vi "GetSwerveEncoders.vi"() -> (20 "Swerve 0 Azimuth Position (deg)":dbl, 21 "Swerve 0 Distance (in)":dbl, 22 "Swerve 1 Azimuth Position (deg)":dbl, 23 "Swerve 1 Distance (in)":dbl, 24 "Swerve 2 Azimuth Position (deg)":dbl, 25 "Swerve 2 Distance (in)":dbl, 26 "Swerve 3 Azimuth Position (deg)":dbl, 27 "Swerve 3 Distance (in)":dbl)   [LabVIEW 2019]
doc: "Gets the drive distance, azimuth position, and velocity encoder readings from the swerve."
uses:
  refnums.vi
  GRNF_POT.vi
  dsdata.vi
  <vilib>/Utility/xml.llb/Write to XML File(string).vi
  outputs.vi
  sensors.vi
  GRNF_CTREMotor.vi
  <vilib>/Rock Robotics/WPI/ThirdParty/Phoenix-LabVIEW/Motor Controller/Get/CTRE_Phoenix_MotorController_GetSelectedSensorData.vi
panel:
  in  "Plot":bool
  out "Drive Encoder Velocities":cluster{dbl, dbl, dbl, dbl}(graph)
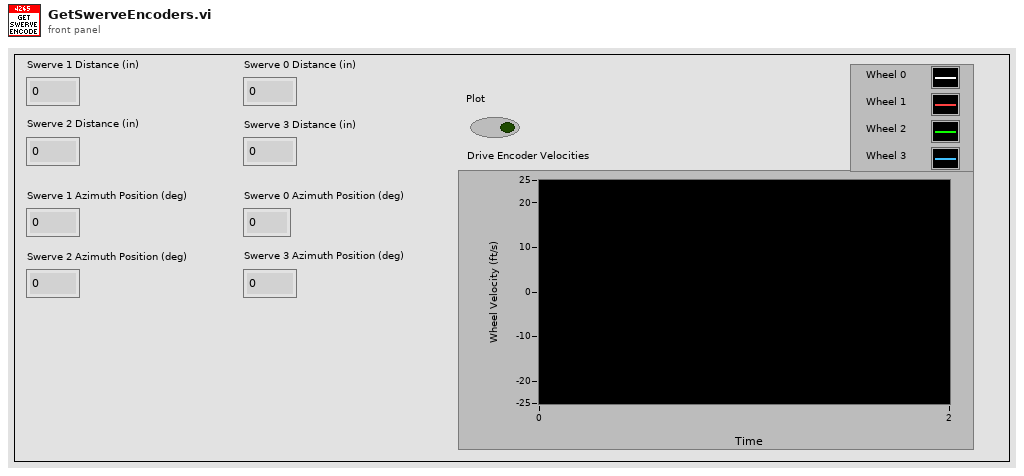
[diagram p1: front panel]
types:
  T1 = typedef "WPI_MotorControlDeviceRef.ctl" = cluster{"DeviceStatus":errorcluster, "Type":T2, "PWM":cluster{"PWM Channel":T3, "DeadBand":T4}, "CAN":cluster{"Device Number":u8, "SetOutput VI Ref":variant, "GetOutput VI Ref":variant, "Enable VI Ref":variant, "Disable VI Ref":variant, "Data":variant}, "Invert":bool, "DIO PWM":cluster{"PWM \"Enable\" Channel":T3, "DIOChannel":T5, "PWM Rate":dbl}}
  T2 = typedef "WPI_MotorControlType.ctl" = enum16{"PWM", "CAN", "DIO PWM"}
  T3 = typedef "FPGA_DIOPWMChannel.ctl" = enum8{"PWM 0", "PWM 1", "PWM 2", "PWM 3", "PWM 4", "PWM 5", "PWM 6", "PWM 7", "PWM 8", "PWM 9", "PWM MXP 0", "PWM MXP 1", "PWM MXP 2", "PWM MXP 3", "PWM MXP 4", "PWM MXP 5", "PWM MXP 6", "PWM MXP 7", "PWM MXP 8", "PWM MXP 9", "Invalid"}
  T4 = typedef "WPI_PWMDeadband.ctl" = cluster{"Name":string, "maxPositivePwm":i32, "minPositivePwm":i32, "centerPwm":i32, "maxNegativePwm":i32, "minNegativePwm":i32, "angularRange":u16}
  T5 = typedef "FPGA_DIOChannel.ctl" = enum8{"DIO 0", "DIO 1", "DIO 2", "DIO 3", "DIO 4", "DIO 5", "DIO 6", "DIO 7", "DIO 8", "DIO 9", "DIO MXP 0", "DIO MXP 1", "DIO MXP 2", "DIO MXP 3", "DIO MXP 4", "DIO MXP 5", "DIO MXP 6", "DIO MXP 7", "DIO MXP 8", "DIO MXP 9", "DIO MXP 10", "DIO MXP 11", "DIO MXP 12", "DIO MXP 13", "DIO MXP 14", "DIO MXP 15", "SPI Port CS1", "SPI Port CS2", "SPI Port CS3", "SPI Port MISO", "SPI Port MOSI", "Invalid"}
  T6 = typedef "WPI_PotentiometerDevRef.ctl" = cluster{"DevStatus":errorcluster, "Analog Channel":T7, "Invert Output":bool}
  T7 = typedef "FPGA_AIChannel.ctl" = enum8{"AI 0", "AI 1", "AI 2", "AI 3", "AI MXP 0", "AI MXP 1", "AI MXP 2", "AI MXP 3", "Invalid"}
  T8 = cluster{"Command Output":bool, "Time Output (ms)":u32}
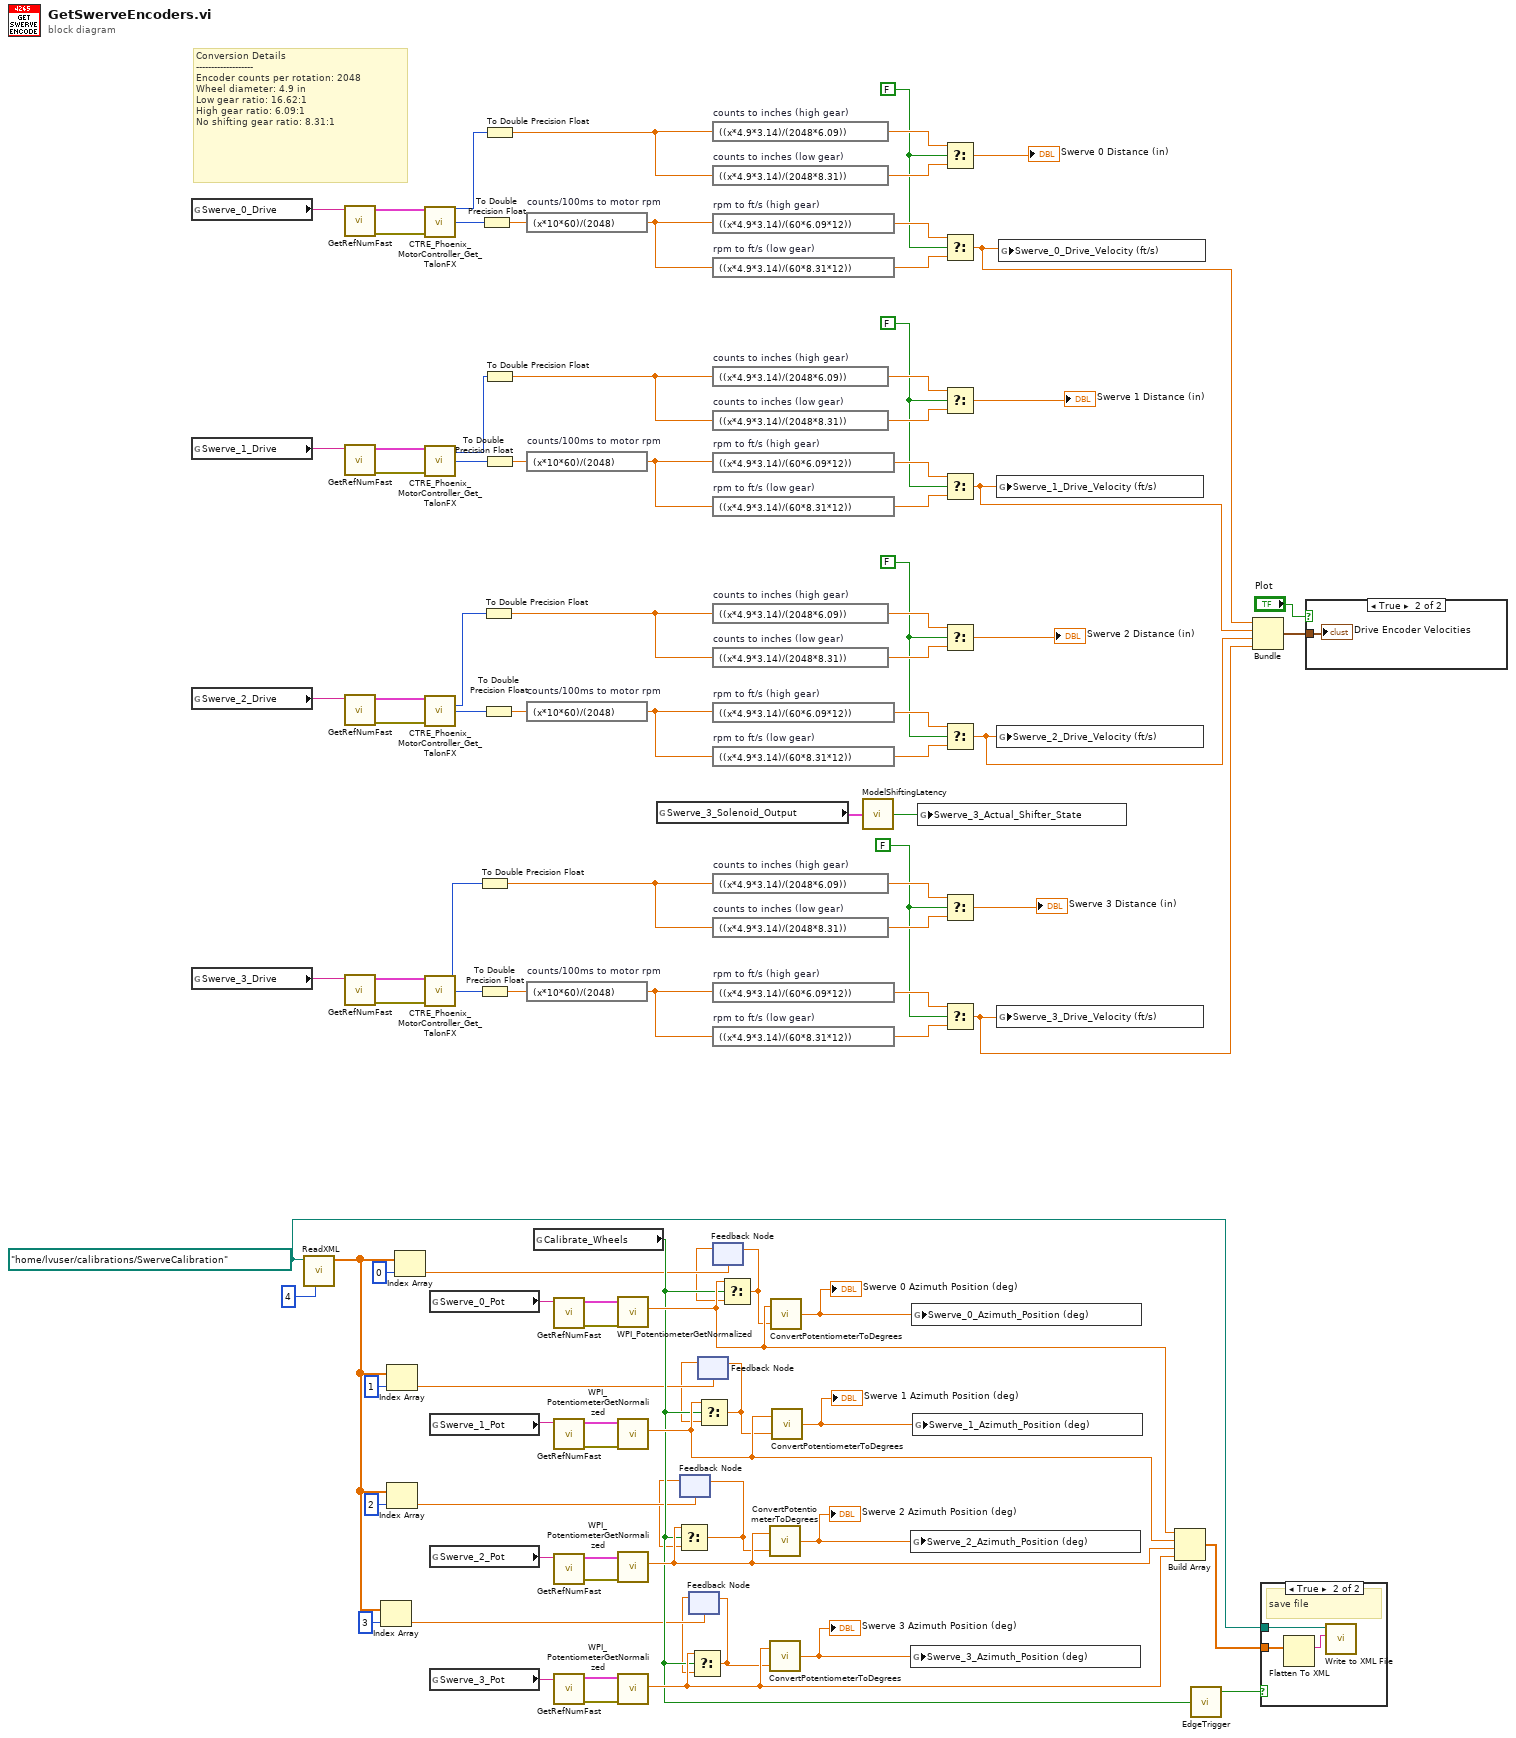
[diagram p0: block diagram]
diagram:
  w13 = FALSE
  w15 = FALSE
  w16 = FALSE
  w17 = FALSE
  w101 = path "/home/lvuser/calibrations/SwerveCalibration" ("path")
  # "Conversion Details\n-------------------\nEncoder counts per rotation: 2048\nWheel diameter: 4.9 in\nLow gear ratio: 16.62:1\nHigh gear ratio: 6.09:1\nNo shifting gear ratio: 8.31:1"
  n1 = global read "refnums.vi" "Swerve_0_Drive"() -> (w25:string)
  n2 = global read "refnums.vi" "Swerve_1_Drive"() -> (w36:string)
  n3 = global read "refnums.vi" "Swerve_2_Drive"() -> (w48:string)
  n4 = global read "refnums.vi" "Swerve_3_Drive"() -> (w58:string)
  n5 = call "ReadXML.vi"("Default Number of Elements"=4 ("Number of Elements"), "File Path (.xml)"=w101) -> ("Data"=w66:dbl[])  [unwired: 8 in, 1 out]
  n6 = call-poly "GetRefNumFast.vi"("RefNum Name"=w25) -> ("Error"=w27:errorcluster, "Device Reference"=w26:T1)  [unwired: 5 in]
  n7 = call-poly "GetRefNumFast.vi"("RefNum Name"=w36) -> ("Error"=w38:errorcluster, "Device Reference"=w37:T1)  [unwired: 5 in]
  n8 = call-poly "GetRefNumFast.vi"("RefNum Name"=w48) -> ("Error"=w50:errorcluster, "Device Reference"=w49:T1)  [unwired: 5 in]
  n9 = call-poly "GetRefNumFast.vi"("RefNum Name"=w58) -> ("Error"=w60:errorcluster, "Device Reference"=w59:T1)  [unwired: 5 in]
  n10 = Index Array(array=w66, index=3) -> (element=w85:dbl)
  n11 = Index Array(array=w66, index=1) -> (element=w90:dbl)
  n12 = Index Array(array=w66, index=2) -> (element=w87:dbl)
  n13 = Index Array(array=w66, index=0) -> (element=w93:dbl)
  n14 = call-poly <vilib>:"CTRE_Phoenix_MotorController_Get_TalonFX.vi"("PhoenixMotorControlDevRef"=w26, "error in"=w27) -> ("Position (Raw Sensor Units)"=w19:i32, "Velocity (Raw Sensor Units per 100 ms)"=w21:i32)  [unwired: 10 in, 2 out]
  n15 = call-poly <vilib>:"CTRE_Phoenix_MotorController_Get_TalonFX.vi"("PhoenixMotorControlDevRef"=w37, "error in"=w38) -> ("Position (Raw Sensor Units)"=w30:i32, "Velocity (Raw Sensor Units per 100 ms)"=w32:i32)  [unwired: 10 in, 2 out]
  n16 = call-poly <vilib>:"CTRE_Phoenix_MotorController_Get_TalonFX.vi"("PhoenixMotorControlDevRef"=w49, "error in"=w50) -> ("Position (Raw Sensor Units)"=w42:i32, "Velocity (Raw Sensor Units per 100 ms)"=w44:i32)  [unwired: 10 in, 2 out]
  n17 = call-poly <vilib>:"CTRE_Phoenix_MotorController_Get_TalonFX.vi"("PhoenixMotorControlDevRef"=w59, "error in"=w60) -> ("Position (Raw Sensor Units)"=w52:i32, "Velocity (Raw Sensor Units per 100 ms)"=w54:i32)  [unwired: 10 in, 2 out]
  n18 = global read "refnums.vi" "Swerve_0_Pot"() -> (w78:string)
  n19 = global read "refnums.vi" "Swerve_1_Pot"() -> (w73:string)
  n20 = global read "refnums.vi" "Swerve_2_Pot"() -> (w70:string)
  n21 = global read "refnums.vi" "Swerve_3_Pot"() -> (w69:string)
  n22 = To Double Precision Float(number=w52) -> (double precision float=w12:dbl)
  n23 = To Double Precision Float(number=w54) -> (double precision float=w11:dbl)
  n24 = To Double Precision Float(number=w21) -> (double precision float=w5:dbl)
  n25 = To Double Precision Float(number=w42) -> (double precision float=w10:dbl)
  n26 = To Double Precision Float(number=w44) -> (double precision float=w9:dbl)
  n27 = To Double Precision Float(number=w19) -> (double precision float=w6:dbl)
  n28 = To Double Precision Float(number=w30) -> (double precision float=w8:dbl)
  n29 = To Double Precision Float(number=w32) -> (double precision float=w7:dbl)
  n30 = expression code="(x*10*60)/(2048)" "counts/100ms to motor rpm"(w5) -> (w28:dbl)
  n31 = expression code="(x*10*60)/(2048)" "counts/100ms to motor rpm"(w7) -> (w39:dbl)
  n32 = expression code="(x*10*60)/(2048)" "counts/100ms to motor rpm"(w9) -> (w51:dbl)
  n33 = expression code="(x*10*60)/(2048)" "counts/100ms to motor rpm"(w11) -> (w62:dbl)
  n34 = global read "dsdata.vi" "Calibrate_Wheels"() -> (w100:bool)
  n35 = call-poly "GetRefNumFast.vi"("RefNum Name"=w78) -> ("Error"=w76:errorcluster, "Device Reference"=w77:T6)  [unwired: 5 in]
  n36 = call-poly "GetRefNumFast.vi"("RefNum Name"=w73) -> ("Error"=w74:errorcluster, "Device Reference"=w75:T6)  [unwired: 5 in]
  n37 = call-poly "GetRefNumFast.vi"("RefNum Name"=w70) -> ("Error"=w71:errorcluster, "Device Reference"=w72:T6)  [unwired: 5 in]
  n38 = call-poly "GetRefNumFast.vi"("RefNum Name"=w69) -> ("Error"=w67:errorcluster, "Device Reference"=w68:T6)  [unwired: 5 in]
  n39 = call <vilib>:"WPI_PotentiometerGetNormalized.vi"("error in"=w76, "PotDevRef"=w77) -> ("Normalized Value"=w102:dbl)  [unwired: 7 in, 2 out]
  n40 = call <vilib>:"WPI_PotentiometerGetNormalized.vi"("error in"=w74, "PotDevRef"=w75) -> ("Normalized Value"=w105:dbl)  [unwired: 7 in, 2 out]
  n41 = call <vilib>:"WPI_PotentiometerGetNormalized.vi"("error in"=w71, "PotDevRef"=w72) -> ("Normalized Value"=w104:dbl)  [unwired: 7 in, 2 out]
  n42 = call <vilib>:"WPI_PotentiometerGetNormalized.vi"("error in"=w67, "PotDevRef"=w68) -> ("Normalized Value"=w103:dbl)  [unwired: 7 in, 2 out]
  n43 = global read "outputs.vi" "Swerve_3_Solenoid_Output"() -> (w61:T8)
  n44 = feedback #1(w87) -> (w86:dbl)
  n45 = Select(t=w104, s=w100, f=w86) -> (s? t:f=w80:dbl)
  n46 = feedback-in #1(w80) -> ()
  n47 = feedback #2(w85) -> (w84:dbl)
  n48 = Select(t=w103, s=w100, f=w84) -> (s? t:f=w79:dbl)
  n49 = feedback-in #2(w79) -> ()
  n50 = feedback #3(w90) -> (w89:dbl)
  n51 = Select(t=w105, s=w100, f=w89) -> (s? t:f=w81:dbl)
  n52 = feedback-in #3(w81) -> ()
  n53 = expression code="((x*4.9*3.14)/(2048*6.09))" "counts to inches (high gear)"(w6) -> (w22:dbl)
  n54 = expression code="((x*4.9*3.14)/(2048*8.31))" "counts to inches (low gear)"(w6) -> (w20:dbl)
  n55 = expression code="((x*4.9*3.14)/(60*6.09*12))" "rpm to ft/s (high gear)"(w28) -> (w24:dbl)
  n56 = expression code="((x*4.9*3.14)/(60*8.31*12))" "rpm to ft/s (low gear)"(w28) -> (w23:dbl)
  n57 = expression code="((x*4.9*3.14)/(2048*6.09))" "counts to inches (high gear)"(w8) -> (w33:dbl)
  n58 = expression code="((x*4.9*3.14)/(2048*8.31))" "counts to inches (low gear)"(w8) -> (w31:dbl)
  n59 = expression code="((x*4.9*3.14)/(60*6.09*12))" "rpm to ft/s (high gear)"(w39) -> (w35:dbl)
  n60 = expression code="((x*4.9*3.14)/(60*8.31*12))" "rpm to ft/s (low gear)"(w39) -> (w34:dbl)
  n61 = expression code="((x*4.9*3.14)/(2048*6.09))" "counts to inches (high gear)"(w10) -> (w45:dbl)
  n62 = expression code="((x*4.9*3.14)/(2048*8.31))" "counts to inches (low gear)"(w10) -> (w43:dbl)
  n63 = expression code="((x*4.9*3.14)/(60*6.09*12))" "rpm to ft/s (high gear)"(w51) -> (w47:dbl)
  n64 = expression code="((x*4.9*3.14)/(60*8.31*12))" "rpm to ft/s (low gear)"(w51) -> (w46:dbl)
  n65 = expression code="((x*4.9*3.14)/(2048*6.09))" "counts to inches (high gear)"(w12) -> (w55:dbl)
  n66 = expression code="((x*4.9*3.14)/(2048*8.31))" "counts to inches (low gear)"(w12) -> (w53:dbl)
  n67 = expression code="((x*4.9*3.14)/(60*6.09*12))" "rpm to ft/s (high gear)"(w62) -> (w57:dbl)
  n68 = expression code="((x*4.9*3.14)/(60*8.31*12))" "rpm to ft/s (low gear)"(w62) -> (w56:dbl)
  n69 = feedback #4(w93) -> (w92:dbl)
  n70 = Select(t=w102, s=w100, f=w92) -> (s? t:f=w82:dbl)
  n71 = feedback-in #4(w82) -> ()
  n72 = call "ConvertPotentiometerToDegrees.vi"("Zero Position [0-1]"=w80, "Raw Potentiometer Value [0,1]"=w104) -> ("Orientation (deg) [-180,+180]"=w96:dbl)
  "Swerve 2 Azimuth Position (deg)" <- w96
  n73 = call "ConvertPotentiometerToDegrees.vi"("Zero Position [0-1]"=w79, "Raw Potentiometer Value [0,1]"=w103) -> ("Orientation (deg) [-180,+180]"=w95:dbl)
  "Swerve 3 Azimuth Position (deg)" <- w95
  n74 = call "ConvertPotentiometerToDegrees.vi"("Zero Position [0-1]"=w82, "Raw Potentiometer Value [0,1]"=w102) -> ("Orientation (deg) [-180,+180]"=w98:dbl)
  "Swerve 0 Azimuth Position (deg)" <- w98
  n75 = call "ConvertPotentiometerToDegrees.vi"("Zero Position [0-1]"=w81, "Raw Potentiometer Value [0,1]"=w105) -> ("Orientation (deg) [-180,+180]"=w97:dbl)
  "Swerve 1 Azimuth Position (deg)" <- w97
  n76 = call "ModelShiftingLatency.vi"("Swerve_Solenoid_Output"=w61) -> ("Actual State"=w14:bool)
  n77 = global write "sensors.vi" "Swerve_2_Azimuth_Position (deg)"(w96) -> ()
  n78 = global write "sensors.vi" "Swerve_3_Azimuth_Position (deg)"(w95) -> ()
  n79 = global write "sensors.vi" "Swerve_0_Azimuth_Position (deg)"(w98) -> ()
  n80 = global write "sensors.vi" "Swerve_1_Azimuth_Position (deg)"(w97) -> ()
  n81 = global write "sensors.vi" "Swerve_3_Actual_Shifter_State"(w14) -> ()
  n82 = Select(t=w22, s=w17, f=w20) -> (s? t:f=→"Swerve 0 Distance (in)":dbl)
  n83 = Select(t=w24, s=w17, f=w23) -> (s? t:f=w18:dbl)
  n84 = Select(t=w33, s=w16, f=w31) -> (s? t:f=→"Swerve 1 Distance (in)":dbl)
  n85 = Select(t=w35, s=w16, f=w34) -> (s? t:f=w29:dbl)
  n86 = Select(t=w45, s=w15, f=w43) -> (s? t:f=→"Swerve 2 Distance (in)":dbl)
  n87 = Select(t=w47, s=w15, f=w46) -> (s? t:f=w41:dbl)
  n88 = Select(t=w55, s=w13, f=w53) -> (s? t:f=→"Swerve 3 Distance (in)":dbl)
  n89 = Select(t=w57, s=w13, f=w56) -> (s? t:f=w63:dbl)
  n90 = global write "sensors.vi" "Swerve_1_Drive_Velocity (ft/s)"(w29) -> ()
  n91 = global write "sensors.vi" "Swerve_2_Drive_Velocity (ft/s)"(w41) -> ()
  n92 = global write "sensors.vi" "Swerve_3_Drive_Velocity (ft/s)"(w63) -> ()
  n93 = global write "sensors.vi" "Swerve_0_Drive_Velocity (ft/s)"(w18) -> ()
  n94 = Build Array(w102, w105, w104, w103) -> (w106:dbl[])
  n95 = call "EdgeTrigger.vi"("Input Signal"=w100) -> ("Rising Edge Trigger"=w99:bool)  [unwired: 2 out]
  n96 = Bundle(w18, w29, w41, w63) -> (w40:cluster{dbl, dbl, dbl, dbl})  [unwired: 1 in]
  n97 = case shown="True" w99 {
    tunnel: w101 -> [_ w109]
    tunnel: w106 -> [_ w108]
    frame False {
    }
    frame True {
      # "save file"
      n98 = Flatten To XML(anything=w108) -> (xml string=w107:string)
      n99 = call-poly <vilib>:"Write to XML File.vi"("XML Input"=w107, "XML File Path"=w109) -> ()  [unwired: 7 in, 3 out]
    }
  }
  n100 = case shown="True" "Plot" {
    tunnel: w40 -> [_ w110]
    frame False {
    }
    frame True {
      "Drive Encoder Velocities" <- w110
    }
  }
